vi "Global_ACT Write_Data Out.vi"() -> ()   [LabVIEW 2016, in "WC_Drive.lvlib"]
uses:
  WC_Drive.lvlib
  TypeDef/CLUSTER_Drive_HW_SRX_Status.ctl
  TypeDef/CLUSTER_4296_SRX_Status.ctl
  TypeDef/CLUSTER_SRX_Status Data.ctl
  TypeDef/CLUSTER_SRX_Encoder Data.ctl
  TypeDef/CLUSTER_SRX_PWM Data.ctl
  TypeDef/CLUSTER_SRX_Analog Data.ctl
  TypeDef/CLUSTER_SRX_Limit Switch Data.ctl
  TypeDef/CLUSTER_SRX_Profile Data.ctl
panel:
  in  "WC_Drive_HW_SRX_Status":T1
  # "The Names of the Data items in the Global Variable MUST describe who the Single Writer is\nNaming Convention of all Data Items is:   Lib Name_Loop Name (SM or SEN or ACT)_Data Name\nExample   Drive_ACT_X axis;  GameController_SEN_JoystickLeft;  Hopper_SM_AgitatorSpeed"
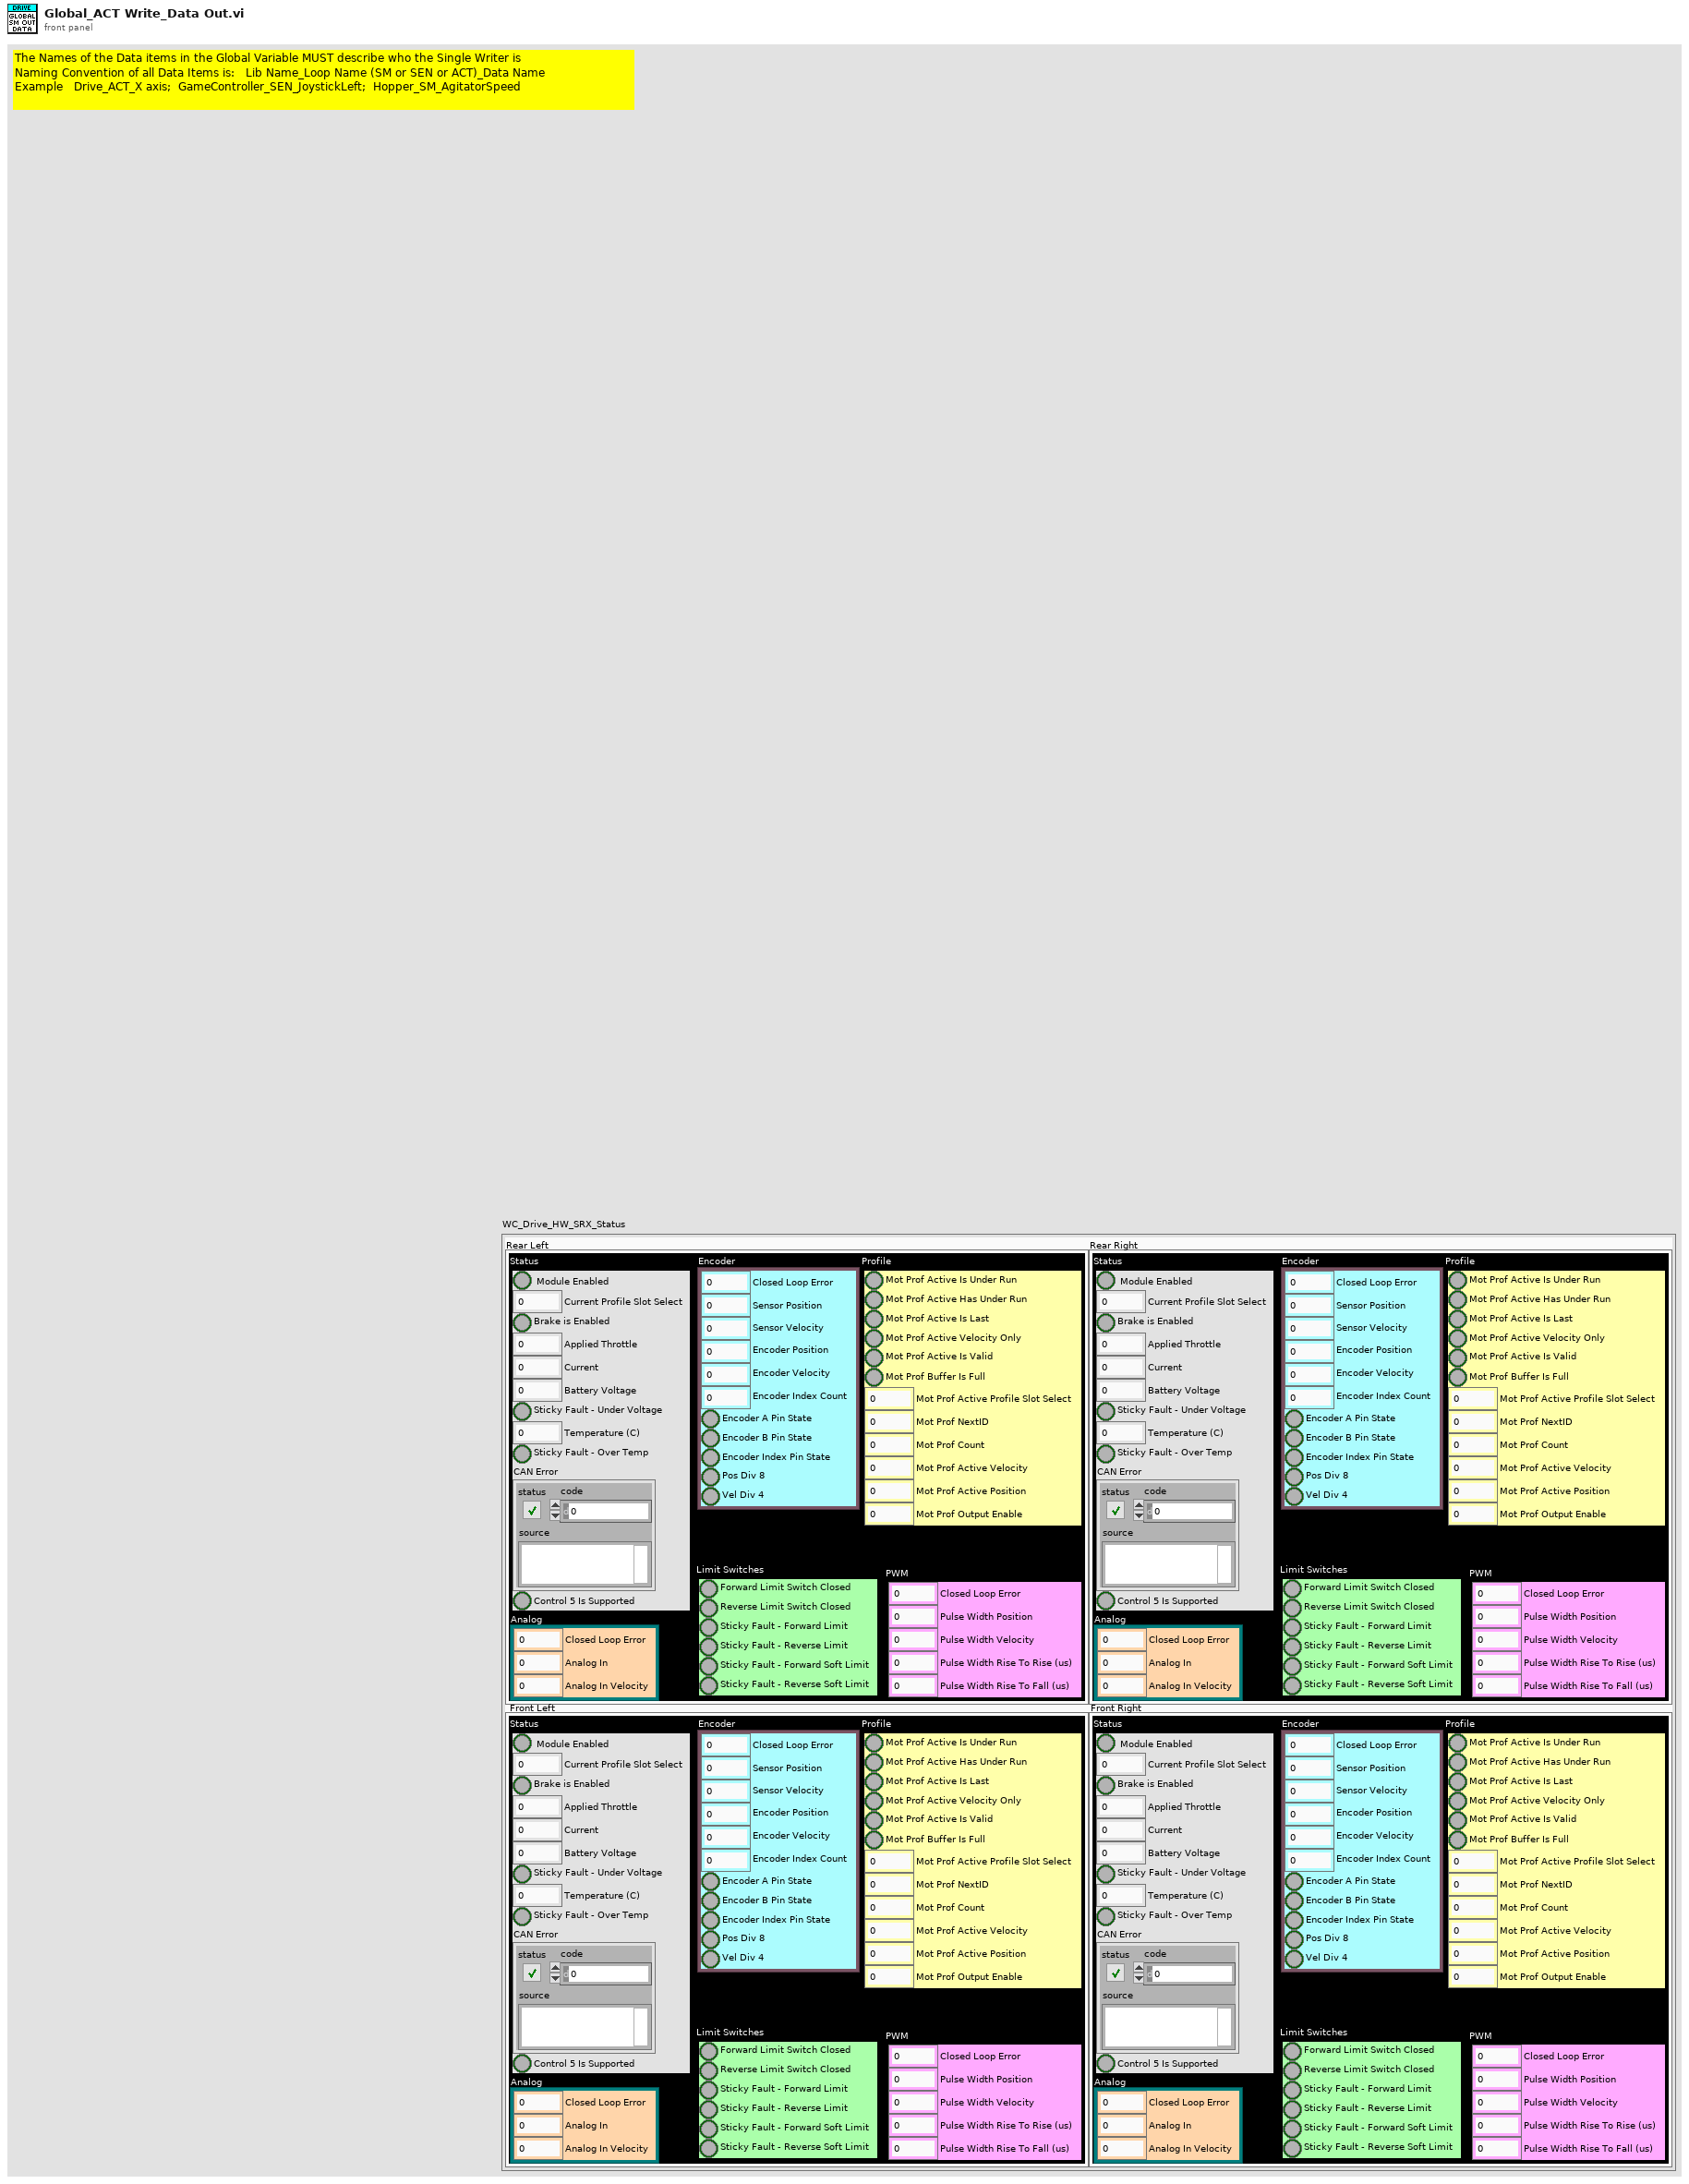
[diagram p1: front panel]
types:
  T1 = typedef "CLUSTER_Drive_HW_SRX_Status.ctl" = cluster{"Rear Left":T2, "Rear Right":T2, "Front Left":T2, "Front Right":T2}
  T2 = typedef "CLUSTER_4296_SRX_Status.ctl" = cluster{"Status":T3, "Encoder":T4, "PWM ":T5, "Analog":T6, "Limit Switches":T7, "Profile":T8}
  T3 = typedef "CLUSTER_SRX_Status Data.ctl" = cluster{"Module Enabled":bool, "Current Profile Slot Select":dbl, "Brake is Enabled":bool, "Applied Throttle":dbl, "Current":dbl, "Battery Voltage":dbl, "Sticky Fault - Under Voltage":bool, "Temperature (C)":dbl, "Sticky Fault - Over Temp":bool, "CAN Error":errorcluster, "Control 5 Is Supported":bool}
  T4 = typedef "CLUSTER_SRX_Encoder Data.ctl" = cluster{"Closed Loop Error":dbl, "Sensor Position":dbl, "Sensor Velocity":dbl, "Encoder Position":dbl, "Encoder Velocity":dbl, "Encoder Index Count":dbl, "Encoder A Pin State":bool, "Encoder B Pin State":bool, "Encoder Index Pin State":bool, "Pos Div 8":bool, "Vel Div 4":bool}
  T5 = typedef "CLUSTER_SRX_PWM Data.ctl" = cluster{"Closed Loop Error":dbl, "Pulse Width Position":i32, "Pulse Width Velocity":i32, "Pulse Width Rise To Rise (us)":i32, "Pulse Width Rise To Fall (us)":i32}
  T6 = typedef "CLUSTER_SRX_Analog Data.ctl" = cluster{"Closed Loop Error":dbl, "Analog In":dbl, "Analog In Velocity":dbl}
  T7 = typedef "CLUSTER_SRX_Limit Switch Data.ctl" = cluster{"Forward Limit Switch Closed":bool, "Reverse Limit Switch Closed":bool, "Sticky Fault - Forward Limit":bool, "Sticky Fault - Reverse Limit":bool, "Sticky Fault - Forward Soft Limit":bool, "Sticky Fault - Reverse Soft Limit":bool}
  T8 = typedef "CLUSTER_SRX_Profile Data.ctl" = cluster{"Mot Prof Active Is Under Run":bool, "Mot Prof Active Has Under Run":bool, "Mot Prof Active Is Last":bool, "Mot Prof Active Velocity Only":bool, "Mot Prof Active Is Valid":bool, "Mot Prof Buffer Is Full":bool, "Mot Prof Active Profile Slot Select":i32, "Mot Prof NextID":i32, "Mot Prof Count":i32, "Mot Prof Active Velocity":dbl, "Mot Prof Active Position":dbl, "Mot Prof Output Enable":i32}
diagram:
